vi "scan info file add preamble.vi"(9 "scan #":string, 10 "device and variable stuff":string, 11 "spreadsheet string":string) -> (3 "scan text for txt file":string)   [LabVIEW 2013]
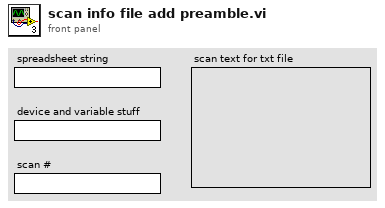
[diagram p1: front panel]
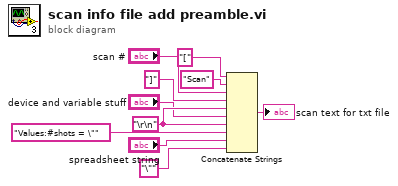
[diagram p0: block diagram]
diagram:
  w9 = "\r\n"
  n1 = Concatenate Strings("[" ("string"), "Scan", "scan #", "]" ("string"), w9, "device and variable stuff", w9, "Values:#shots = \"" ("string"), "spreadsheet string", "\"" ("string")) -> (→"scan text for txt file":string)
